vi "Coil Calib Select and Get.vi"(4 "error in (no error)":errorcluster, 7 "Magnet ID":string) -> (0 "error out":errorcluster, 2 "File Name":string, 3 "String":string)   [LabVIEW 2020]
panel:
  in  "OK":bool
  in  "Cell Name":u16(ring) items=["Cell 12", "Cell 15 Both Ins_Out Coil Fit", "Cell 15 Insert", "Cell 2", "Cell 4", "Cell 5 22T", "Cell 5 25T", "Cell 5", "Cell 6", "Cell 7", "Cell 8", "Cell 9", "None"]
  # "Please Select a Calibration File"
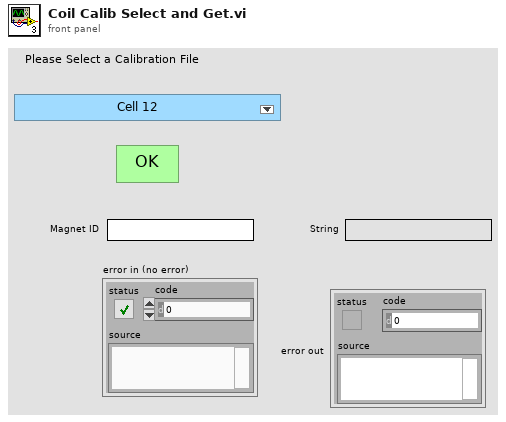
[diagram p1: front panel]
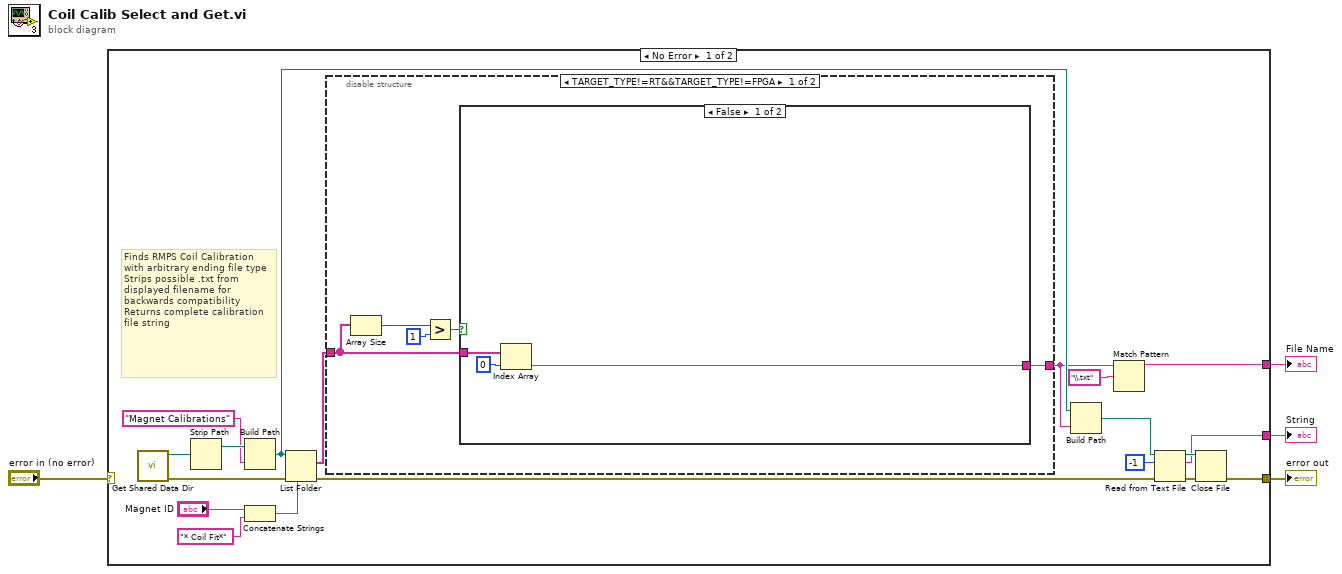
[diagram p0: block diagram]
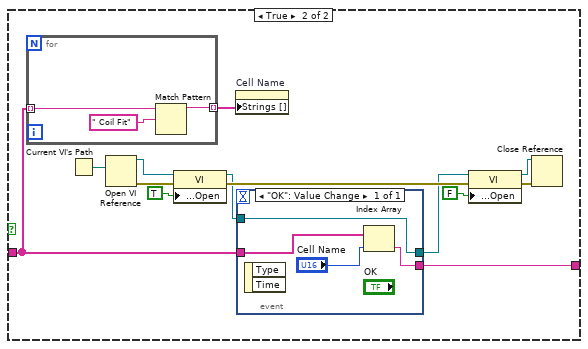
[diagram p2: hidden frame]
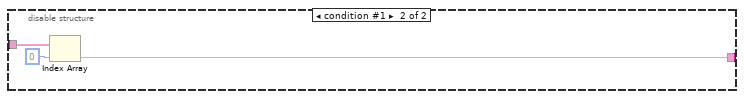
[diagram p3: hidden frame]
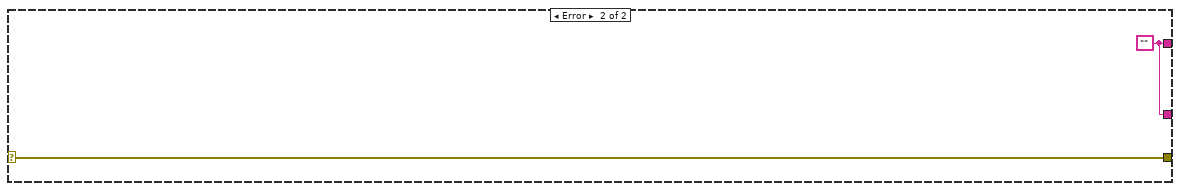
[diagram p4: hidden frame]
diagram:
  n1 = case shown="No Error" "error in (no error)" {
    selector: "error in (no error)" -> [_ w56]
    tunnel: [w19 w55] -> w4
    tunnel: [w10 w56] -> w3
    tunnel: [w7 w55] -> w2
    frame No Error {
      # "Finds RMPS Coil Calibration with arbitrary ending file type\nStrips possible .txt from displayed filename for backwards compatibility\nReturns complete calibration file string"
      n2 = call "Get Shared Data Dir.vi"() -> ("Error Out"=w6:errorcluster, "Data Directory Path"=w16:path)  [unwired: 2 in]
      n3 = Strip Path(path=w16) -> (stripped path=w17:path)  [unwired: 1 out]
      n4 = Build Path(base path=w17, name or relative path="Magnet Calibrations") -> (appended path=w22:path)
      n5 = Concatenate Strings("Magnet ID", "* Coil Fit*") -> (w21:string)
      n6 = List Folder(path=w22, pattern=w21, error in=w6) -> (filenames=w12:string[], error out=w5:errorcluster)  [unwired: 1 in, 2 out]
      n7 = disable-structure shown="TARGET_TYPE!=RT&&TARGET_TYPE!=FPGA" {
        disable-tunnel: w12 -> [w28 w53]
        disable-tunnel: [w24 w52] -> w9
        frame condition #0 (active) {
          n8 = Array Size(array=w28) -> (size(s)=w27:i32)
          n9 = Greater?(x=w27, y=1) -> (0:w25:bool)
          n10 = case shown="False" w25 {
            tunnel: [w31 w36] -> w24
            tunnel: w28 -> [w30 w33]
            frame False {
              n11 = Index Array(array=w30, index=0) -> (element=w31:string)
            }
            frame True {
              n12 = for {
                tunnel: w33 -> [w47] mode=indexing
                tunnel: [w45] -> w32 mode=indexing
                n13 = Match Pattern(string=w47, regular expression=" Coil Fit") -> (before substring=w45:string)  [unwired: 1 in, 3 out]
              }
              n14 = Current VI's Path() -> (path=w44:path)
              n15 = Open VI Reference(vi path=w44) -> (vi reference=w43:refnum<vi>, error out=w38:errorcluster)  [unwired: 5 in]
              n16 = property class="VI"(reference=w43, error in=w38, "Front Panel.Open"=TRUE ("Front Panel Window:Open")) -> (reference out=w34:refnum<vi>, error out=w39:errorcluster)
              n17 = property on="Cell Name" class="Ring (strict)"("Strings []"=w32) -> ()  [unwired: 2 in, 2 out]
              n18 = event shown="[0] \"OK\": Value Change" {
                selector: _ -> [_]
                dyn-events: _ -> [_]
                timeout: _ -> [_]
                tunnel: [w50] -> w36
                tunnel: w33 -> [w49]
                tunnel: [w48] -> w35
                tunnel: w34 -> [w48]
                event "OK": Value Change {
                  n19 = event-data() -> ()  [unwired: 1 in, 2 out]
                  n20 = Index Array(array=w49, index="Cell Name") -> (element=w50:string)
                }
              }
              n21 = property class="VI"(reference=w35, error in=w39, "Front Panel.Open"=FALSE ("Front Panel Window:Open")) -> (reference out=w40:refnum<vi>, error out=w41:errorcluster)
              n22 = Close Reference(reference=w40, error in (no error)=w41) -> ()  [unwired: 1 out]
            }
          }
        }
        frame condition #1 {
          n23 = Index Array(array=w53, index=0) -> (element=w52:string)
        }
      }
      n24 = Build Path(base path=w22, name or relative path=w9) -> (appended path=w23:path)
      n25 = Match Pattern(string=w9, regular expression="\\.txt") -> (before substring=w7:string)  [unwired: 1 in, 3 out]
      n26 = Read from Text File(file (use dialog)=w23, count=-1, error in=w5) -> (refnum out=w20:refnum<file>, text=w19:string, error out=w11:errorcluster)  [unwired: 1 in, 1 out]
      n27 = Close File(refnum=w20, error in=w11) -> (error out=w10:errorcluster)  [unwired: 1 out]
    }
    frame Error {
      w55 = ""
    }
  }
  "error out" <- w3
  "String" <- w4
  "File Name" <- w2
